vi "Configure ARB Sequence Udefined Dwell.vi"(8 "error in":errorcluster, 9 "Dwell(S)":dbl min=0.0, 10 "Step":i32=1 min=1 max=200, 11 "VISA resource name":refnum<visa-resource-name>) -> (0 "error out":errorcluster, 3 "VISA resource name out":refnum<visa-resource-name>)   [LabVIEW 2015, in "IT-M3900C.lvlib"]
doc: "This command sets the time width of the first step in the sequence.\n<b>Step</b>\n1-200\n<b>Dwell(S)</b>\nMIN-MAX"
uses:
  <instrlib>/IT-M3900C/IT-M3900C.lvlib
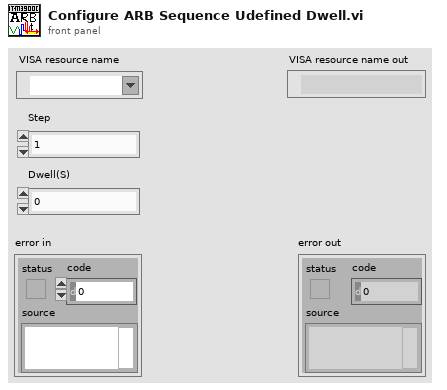
[diagram p1: front panel]
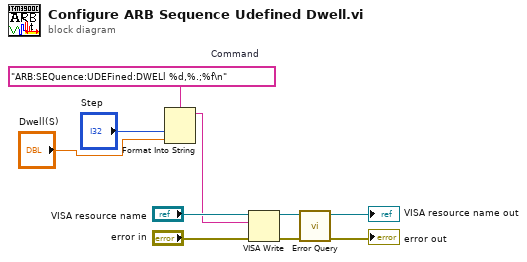
[diagram p0: block diagram]
diagram:
  w4 = "ARB:SEQuence:UDEFined:DWELl %d,%.;%f\n"  # Command
  n1 = Format Into String(format string=w4, "Step", "Dwell(S)") -> (resulting string=w2:string)  [unwired: 2 in, 1 out]
  n2 = VISA Write(VISA resource name="VISA resource name", write buffer=w2, error in (no error)="error in") -> (VISA resource name out=w7:refnum<visa-resource-name>, error out=w8:errorcluster)  [unwired: 1 out]
  n3 = call <instrlib>:"Error Query.vi"("error in"=w8, "VISA resource name"=w7) -> ("error out"=→"error out":errorcluster, "VISA resource name out"=→"VISA resource name out":refnum<visa-resource-name>)  [unwired: 6 in, 2 out]
